vi "ActivateMasterEncoderMode.vi"(4 "error in (no error)":errorcluster, 6 "master encoder parameter":T1, 7 "axis in":cluster{"keyHandle":u32, "nodeId":u16}={"keyHandle"=0, "nodeId"=1}) -> (0 "error out":errorcluster, 3 "axis out":cluster{"keyHandle":u32, "nodeId":u16}={"keyHandle"=0, "nodeId"=1})   [LabVIEW 2017, in "maxonEPOS.lvlib"]
doc: "<B>ActivateMasterEncoderMode</B> changes the operational mode to master encoder mode (MEM)."
uses:
  Examples/maxonEPOS.lvlib
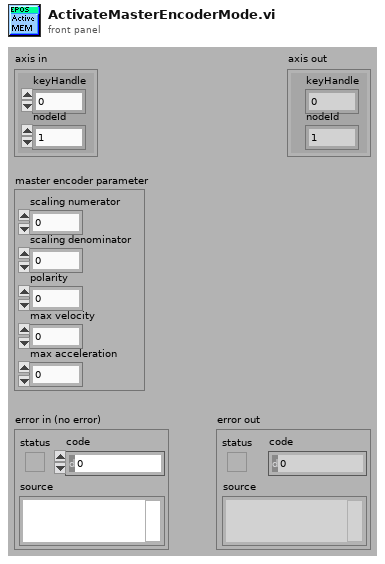
[diagram p1: front panel]
types:
  T1 = cluster{"scaling numerator":u16, "scaling denominator":u16, "polarity":u8, "max velocity":u32, "max acceleration":u32}
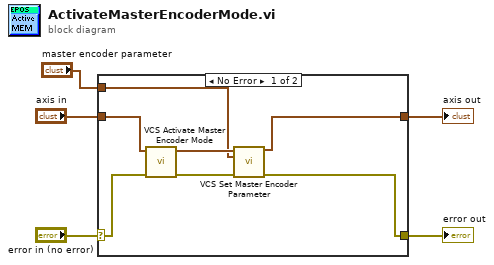
[diagram p0: block diagram]
diagram:
  n1 = case shown="No Error" "error in (no error)" {
    selector: "error in (no error)" -> [w12 w14]
    tunnel: [w7 w14] -> w4
    tunnel: [w8 w13] -> w3
    tunnel: "axis in" -> [w11 w13]
    tunnel: "master encoder parameter" -> [w6 _]
    frame No Error {
      n2 = call "VCS Activate Master Encoder Mode.vi"("error in (no error)"=w12, "axis in"=w11) -> ("error out"=w10:errorcluster, "axis out"=w9:cluster{"keyHandle":u32, "nodeId":u16})  [unwired: 8 in]
      n3 = call "VCS Set Master Encoder Parameter.vi"("axis in"=w9, "master encoder parameter"=w6, "error in (no error)"=w10) -> ("axis out"=w8:cluster{"keyHandle":u32, "nodeId":u16}, "error out"=w7:errorcluster)  [unwired: 11 in]
    }
    frame Error {
    }
  }
  "error out" <- w4
  "axis out" <- w3
